vi "get_curr_valve.vi"(8 "error in (no error)":errorcluster, 11 "VALVE PORT IN":refnum<visa-resource-name>) -> (0 "error out":errorcluster, 2 "Current Valve":i32, 3 "VALVE PORT OUT":refnum<visa-resource-name>)   [LabVIEW 2013]
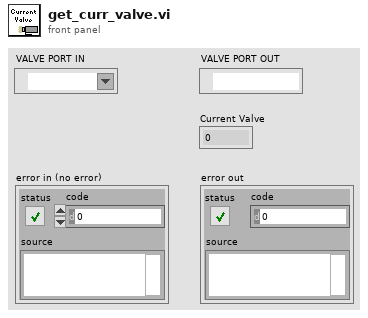
[diagram p1: front panel]
types:
  T1 = enum16{"Move to Home", "Set Positions", "Set Actuator Mode", "OTHER", "Set Direction", "CW Move", "CCW Move"}
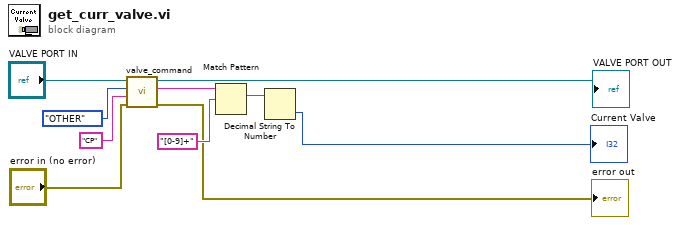
[diagram p0: block diagram]
diagram:
  n1 = call "valve_command.vi"("Error IN"="error in (no error)", "Command option"="CP", "COMMANDS"=T1."OTHER", "VALVE PORT IN"="VALVE PORT IN") -> ("Error OUT"=→"error out":errorcluster, "read buffer"=w3:string, "VALVE PORT OUT"=→"VALVE PORT OUT":refnum<visa-resource-name>)  [unwired: 5 in]
  n2 = Match Pattern(string=w3, regular expression="[0-9]+") -> (match substring=w10:string)  [unwired: 1 in, 3 out]
  n3 = Decimal String To Number(string=w10) -> (number=→"Current Valve":i32)  [unwired: 2 in, 1 out]
